vi "CSM - Filter Messages to Non-Existing Modules.vi"(5 "States In":string) -> (6 "States Out":string)   [LabVIEW 2017, in "Communicable State Machine.lvlib"]
doc: "Filters messages sent to non-existing modules in the CSM state queue. This VI uses the CSM - List Modules VI to obtain all active CSM modules and then filters out messages sent to modules that do not exist.\n\n\n> [!NOTE] <b>CSM State Queue Operation API</b>\n>\n> This type of API only concatenates message strings and does not send messages directly. The message is sent and the operation executed within the Parse State Queue++ VI. Unlike the Message Building API, this type of API includes a CSM state queue string input, which is equivalent to inserting a message into the state queue.\n\n\n-- <b>Controls</b> --\n- <b>States In</b>: The entire state description string to filter.\n\n-- <b>Indicators</b> --\n- <b>States Out</b>: The filtered state description string."
uses:
  Communicable State Machine.lvlib
  _Shared/CSM Shared.lvlib
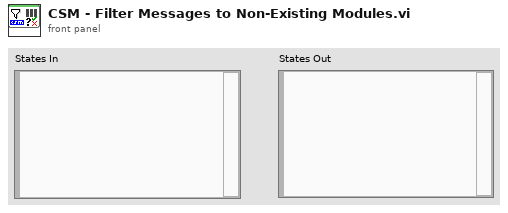
[diagram p1: front panel]
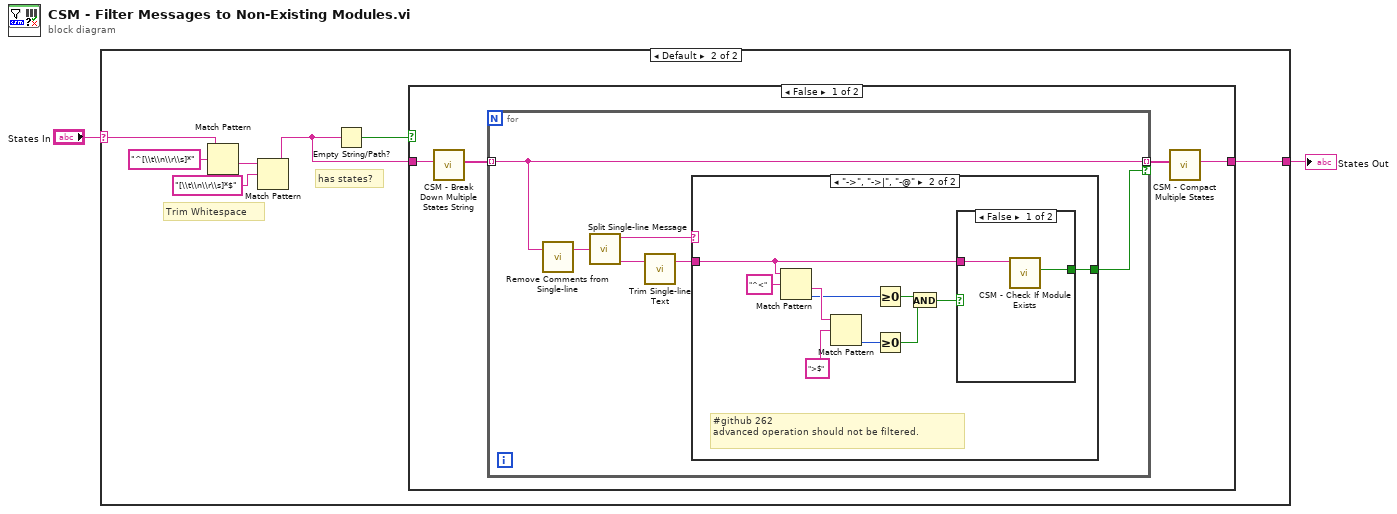
[diagram p0: block diagram]
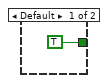
[diagram p3: hidden frame]
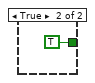
[diagram p4: hidden frame]
diagram:
  n1 = case shown="Default" "States In" {
    selector: "States In" -> [_ w6]
    tunnel: [_ w4] -> w1
    frame "" {
    }
    frame Default {
      # "Trim Whitespace"
      # "has states?"
      n2 = Match Pattern(string=w6, regular expression="^[\\t\\n\\r\\s]*") -> (after substring=w8:string)  [unwired: 1 in, 3 out]
      n3 = Match Pattern(string=w8, regular expression="[\\t\\n\\r\\s]*$") -> (before substring=w5:string)  [unwired: 1 in, 3 out]
      n4 = Empty String/Path?(string/path=w5) -> (empty?=w3:bool)
      n5 = case shown="False" w3 {
        tunnel: w5 -> [w13 w34]
        tunnel: [w12 w34] -> w4
        frame False {
          n6 = call "CSM - Break Down Multiple States String.vi"("States"=w13) -> ("Multiple States"=w11:string[])  [unwired: 10 in]
          n7 = for {
            tunnel: w11 -> [w18] mode=indexing
            tunnel: [w18] -> w10 mode=indexing if=w16
            n8 = call "Remove Comments from Single-line.vi"("single-line text"=w18) -> ("single-line text without comments"=w19:string)  [unwired: 2 in]
            n9 = call "Split Single-line Message.vi"("single-line text"=w19) -> ("operator"=w17:string, "source/target"=w15:string)  [unwired: 6 in, 2 out]
            n10 = call "Trim Single-line Text.vi"("single-line text"=w15) -> ("trimed text"=w14:string)  [unwired: 2 in]
            n11 = case shown="\"->\", \"->|\", \"-@\"" w17 {
              tunnel: [TRUE w30] -> w16
              tunnel: w14 -> [_ w26]
              frame Default {
              }
              frame "->", "->|", "-@" {
                # "#github 262\nadvanced operation should not be filtered."
                n12 = Match Pattern(string=w26, regular expression="^<") -> (after substring=w28:string, offset past match=w25:i32)  [unwired: 1 in, 2 out]
                n13 = Match Pattern(string=w28, regular expression=">$") -> (offset past match=w24:i32)  [unwired: 1 in, 3 out]
                n14 = Greater Or Equal To 0?(x=w25) -> (x >= 0?=w23:bool)
                n15 = Greater Or Equal To 0?(x=w24) -> (x >= 0?=w22:bool)
                n16 = And(x=w23, y=w22) -> (x .and. y?=w21:bool)
                n17 = case shown="False" w21 {
                  tunnel: [w32 TRUE ("Exist?")] -> w30
                  tunnel: w26 -> [w31 _]
                  frame False {
                    n18 = call "CSM - Check If Module Exists.vi"("CSM Name"=w31) -> ("Exist?"=w32:bool)  [unwired: 8 in, 2 out]
                  }
                  frame True {
                  }
                }
              }
            }
          }
          n19 = call "CSM - Compact Multiple States.vi"("Multiple States"=w10) -> ("States"=w12:string)  [unwired: 9 in]
        }
        frame True {
        }
      }
    }
  }
  "States Out" <- w1
